vi "ss_mm calculation in string.vi"(8 "error in (no error)":errorcluster, 9 "Table 2":string[](array[string]), 10 "Table":string[](array[string]), 11 "Numeric":i32) -> (0 "error out":errorcluster, 3 "Array 2":string[](array[string]))   [LabVIEW 2017]
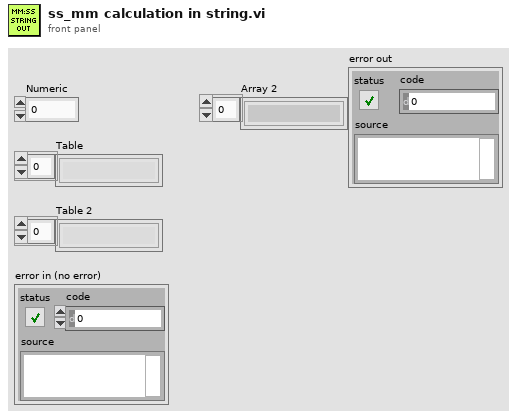
[diagram p1: front panel]
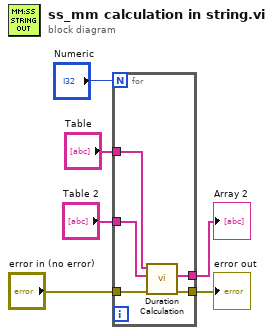
[diagram p0: block diagram]
diagram:
  n1 = for {
    N: "Numeric" -> [_]
    tunnel: "Table 2" -> [w9]
    tunnel: "Table" -> [w10]
    tunnel: [w7] -> w1
    tunnel: "error in (no error)" -> [w8]
    tunnel: [w11] -> w3
    n2 = call "Duration Calculation.vi"("error in (no error)"=w8, "Breakdown out time"=w9, "Breakdown in time"=w10) -> ("error out"=w7:errorcluster, "Array 2"=w11:string[])  [unwired: 5 in, 2 out]
  }
  "Array 2" <- w3
  "error out" <- w1
